vi "DS4Monitor.GetButtonInput.vi"(1 "button info":T2) -> (0 "DS4 Button Input":T1)   [LabVIEW 2024]
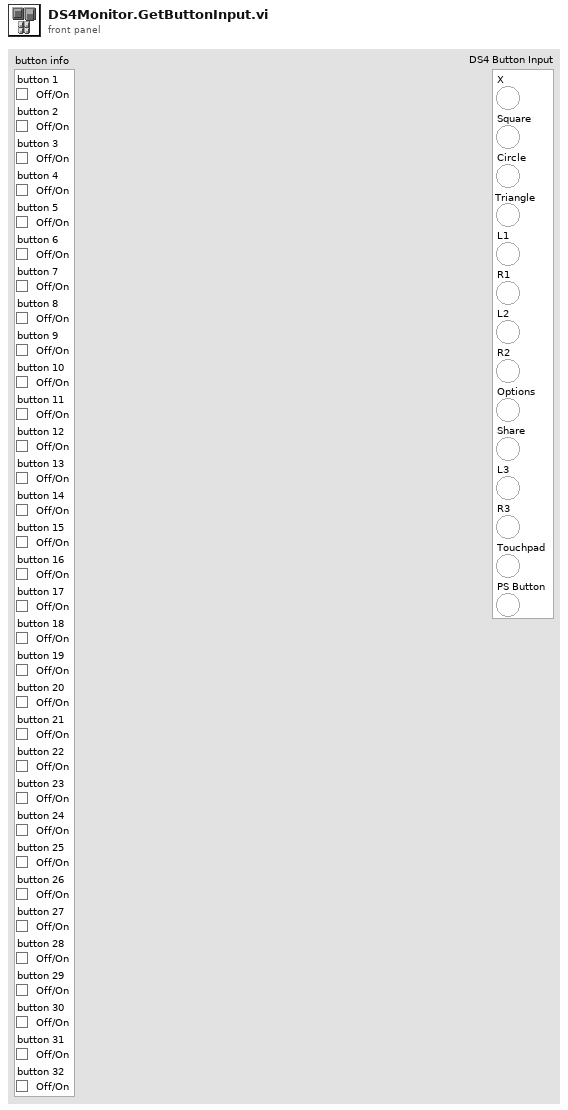
[diagram p1: front panel]
types:
  T1 = cluster{"X":bool, "Square":bool, "Circle":bool, "Triangle":bool, "L1":bool, "R1":bool, "L2":bool, "R2":bool, "Options":bool, "Share":bool, "L3":bool, "R3":bool, "Touchpad":bool, "PS Button":bool}
  T2 = cluster{"button 1":bool, "button 2":bool, "button 3":bool, "button 4":bool, "button 5":bool, "button 6":bool, "button 7":bool, "button 8":bool, "button 9":bool, "button 10":bool, "button 11":bool, "button 12":bool, "button 13":bool, "button 14":bool, "button 15":bool, "button 16":bool, "button 17":bool, "button 18":bool, "button 19":bool, "button 20":bool, "button 21":bool, "button 22":bool, "button 23":bool, "button 24":bool, "button 25":bool, "button 26":bool, "button 27":bool, "button 28":bool, "button 29":bool, "button 30":bool, "button 31":bool, "button 32":bool}
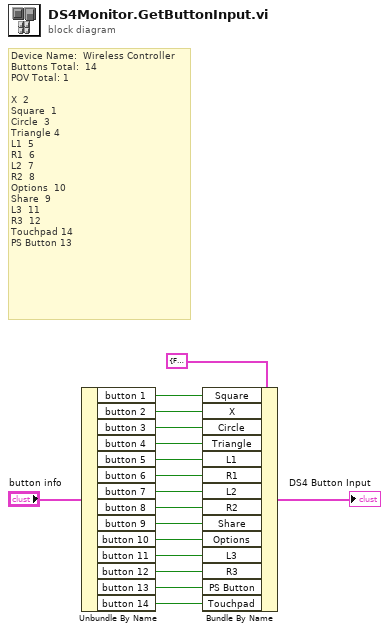
[diagram p0: block diagram]
diagram:
  # "Device Name: \tWireless Controller\nButtons Total: \t14\nPOV Total:\t1\n\nX\t\t2\nSquare\t\t1\nCircle\t\t3\nTriangle\t4\nL1\t\t5\nR1\t\t6\nL2\t\t7\nR2\t\t8\nOptions\t\t10\nShare\t\t9\nL3\t\t11\nR3\t\t12\nTouchpad\t14\nPS Button\t13"
  n1 = Unbundle By Name("button info") -> ("button 1"=w14:bool, "button 2"=w15:bool, "button 3"=w13:bool, "button 4"=w12:bool, "button 5"=w11:bool, "button 6"=w10:bool, "button 7"=w9:bool, "button 8"=w8:bool, "button 9"=w7:bool, "button 10"=w6:bool, "button 11"=w5:bool, "button 12"=w4:bool, "button 13"=w3:bool, "button 14"=w2:bool)
  n2 = Bundle By Name(cluster=T1 {"X"=FALSE, "Square"=FALSE, "Circle"=FALSE, "Triangle"=FALSE, "L1"=FALSE, "R1"=FALSE, "L2"=FALSE, "R2"=FALSE, "Options"=FALSE, "Share"=FALSE, "L3"=FALSE, "R3"=FALSE, "Touchpad"=FALSE, "PS Button"=FALSE}, "Square"=w14, "X"=w15, "Circle"=w13, "Triangle"=w12, "L1"=w11, "R1"=w10, "L2"=w9, "R2"=w8, "Share"=w7, "Options"=w6, "L3"=w5, "R3"=w4, "PS Button"=w3, "Touchpad"=w2) -> (→"DS4 Button Input":T1)
